vi "MGI MGI Max & Min (non-negative) DBL.vi"(2 "y":dbl, 3 "x":dbl) -> (0 "Min Non-Negative":dbl, 1 "Max Non-Negative":dbl)   [LabVIEW 2016]
doc: "Returns the maximum and minimum values among the non-negative inputs. If both of the inputs are negative, then the outputs are both NaN.\n\nAuthored by Thomas E. Henage\nsupport@mooregoodideas.com\nwww.mooregoodideas.com\n\nCopyright (c) 2010, Moore Good Ideas, Inc.\n\nAll rights reserved.\n\nRedistribution and use in source and binary forms, with or without modification, are permitted provided that the following conditions are met:\n\n * Redistributions of source code must retain the above copyright notice, this list of conditions and the following disclaimer.\n * Redistributions in binary form must reproduce the above copyright notice, this list of conditions and the following disclaimer in the documentation and/or other materials provided with the distribution.\n * Neither the name of Moore Good Ideas, Inc. nor the names of its contributors may be used to endorse or promote products derived from this software without specific prior written permission.\n\nTHIS SOFTWARE IS PROVIDED BY THE COPYRIGHT HOLDERS AND CONTRIBUTORS \"AS IS\" AND ANY EXPRESS OR IMPLIED WARRANTIES, INCLUDING, BUT NOT LIMITED TO, THE IMPLIED WARRANTIES OF MERCHANTABILITY AND FITNESS FOR A PARTICULAR PURPOSE ARE DISCLAIMED. IN NO EVENT SHALL THE COPYRIGHT OWNER OR CONTRIBUTORS BE LIABLE FOR ANY DIRECT, INDIRECT, INCIDENTAL, SPECIAL, EXEMPLARY, OR CONSEQUENTIAL DAMAGES (INCLUDING, BUT NOT LIMITED TO, PROCUREMENT OF SUBSTITUTE GOODS OR SERVICES; LOSS OF USE, DATA, OR PROFITS; OR BUSINESS INTERRUPTION) HOWEVER CAUSED AND ON ANY THEORY OF LIABILITY, WHETHER IN CONTRACT, STRICT LIABILITY, OR TORT (INCLUDING NEGLIGENCE OR OTHERWISE) ARISING IN ANY WAY OUT OF THE USE OF THIS SOFTWARE, EVEN IF ADVISED OF THE POSSIBILITY OF SUCH DAMAGE."
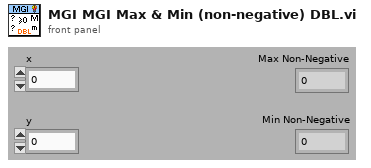
[diagram p1: front panel]
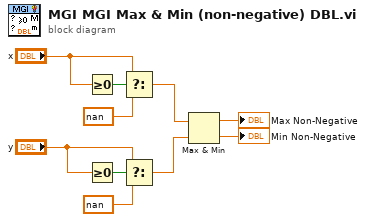
[diagram p0: block diagram]
diagram:
  n1 = Greater Or Equal To 0?(x="x") -> (x >= 0?=w10:bool)
  n2 = Greater Or Equal To 0?(x="y") -> (x >= 0?=w6:bool)
  n3 = Select(t="x", s=w10, f=nan) -> (s? t:f=w4:dbl)
  n4 = Select(t="y", s=w6, f=nan) -> (s? t:f=w3:dbl)
  n5 = Max & Min(x=w4, y=w3) -> (max(x,y)=→"Max Non-Negative":dbl, min(x,y)=→"Min Non-Negative":dbl)
